vi "sub_PSKMod (User).vi"(0 "Packet to Transmit":i8[](array[numeric]), 2 "PSK system parameters":T2 {"PSK type" items=["normal", "shifted", "offset"]; "symbol map" format="%.3f"}, 7 "Symbol Rate, Hz":dbl=1.0 format="%.2f", 11 "error in (no error)":errorcluster, 12 "filter parameters":T1={"Alpha"=0.5, "Filter Length"=6, "TX Filter"=enum."Root Raised Cos"} {"Alpha" format="%.2f"}) -> (4 "output complex waveform":cluster{"t0":dbl, "dt":dbl, "Y":cdb[]} {"Y" format="%.3f"; "dt" format="%^.2e"; "t0" format="%.4f"}, 8 "samples per symbol":i32, 15 "error out":errorcluster)   [LabVIEW 2013]
uses:
  <vilib>/addons/Modulation/niDMT.lvlib
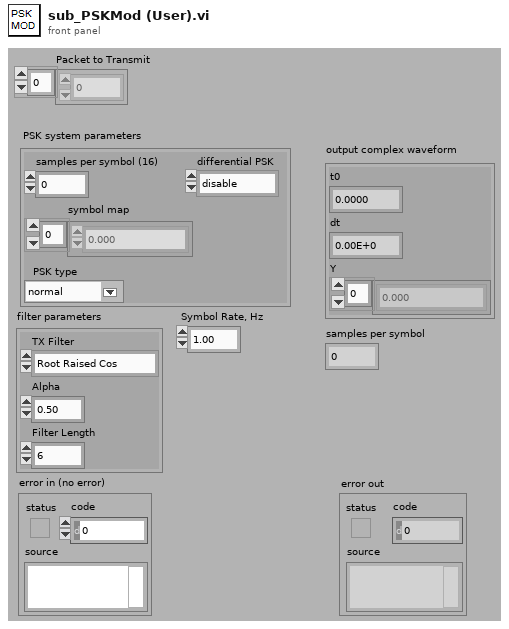
[diagram p1: front panel]
types:
  T1 = cluster{"Alpha":dbl, "Filter Length":i32, "TX Filter":enum16{"none", "Raised Cosine", "Root Raised Cos", "Gaussian"}}
  T2 = cluster{"samples per symbol (16)":i32, "symbol map":cdb[], "differential PSK":enum16{"disable", "enable"}, "PSK type":u16}
  T3 = enum16{"FSK", "PSK", "QAM", "MSK", "PAM", "ASK", "CPM"}
  T4 = enum16{"none", "Raised Cosine", "Root Raised Cos", "Gaussian"}
  T5 = typedef "niAMT.lvlib/Complex Data Waveform.ctl" = cluster{"t0":dbl, "dt":dbl, "Y":cdb[]}
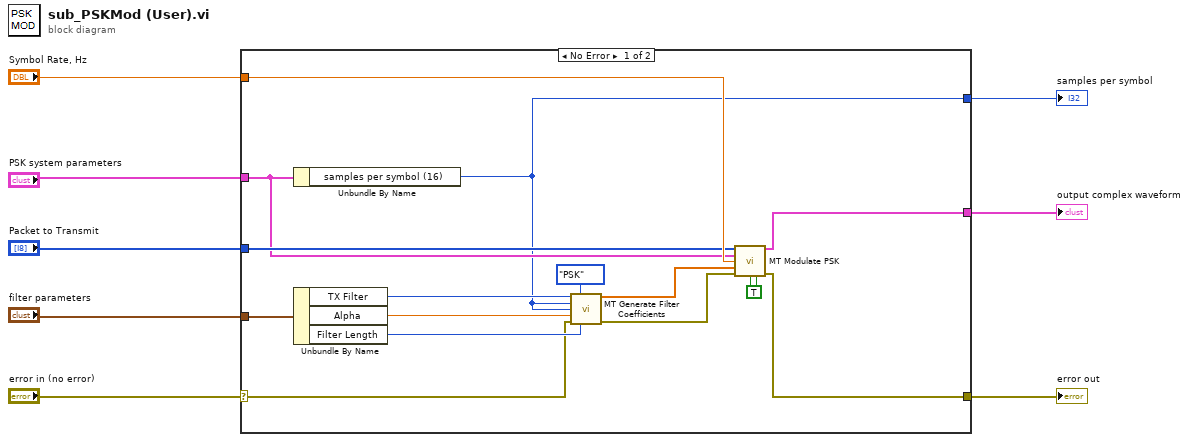
[diagram p0: block diagram]
diagram:
  n1 = case shown="No Error" "error in (no error)" {
    selector: "error in (no error)" -> [w14 w24]
    tunnel: "Symbol Rate, Hz" -> [w22 _]
    tunnel: "PSK system parameters" -> [w12 _]
    tunnel: "filter parameters" -> [w21 _]
    tunnel: "Packet to Transmit" -> [w16 _]
    tunnel: [w11 _] -> w3
    tunnel: [w10 _] -> w2
    tunnel: [w9 w24] -> w1
    frame No Error {
      w23 = TRUE ("Reset (T)")
      n2 = Unbundle By Name(w12) -> ("samples per symbol (16)"=w10:i32)
      n3 = Unbundle By Name(w21) -> ("TX Filter"=w17:T4, "Alpha"=w18:dbl, "Filter Length"=w19:i32)
      n4 = call <vilib>:"MT Generate Filter Coefficients.vi"("pulse shaping filter (none)"=w17, "modulation type"=T3."PSK", "pulse shaping samples per symbol (16)"=w10, "matched samples per symbol (16)"=w10, "filter parameter"=w18, "error in (no error)"=w14, "filter length (symbols)"=w19) -> ("pulse shaping filter coefficients"=w15:dbl[], "error out"=w13:errorcluster)  [unwired: 6 in, 1 out]
      n5 = call <vilib>:"MT Modulate PSK.vi"("input bit stream"=w16, "PSK system parameters"=w12, "symbol rate (Hz)"=w22, "pulse shaping filter coefficients"=w15, "error in (no error)"=w13, "reset? (T)"=w23, "flush buffers? (F)"=w23) -> ("output complex waveform"=w11:T5, "error out"=w9:errorcluster)  [unwired: 6 in, 1 out]
    }
    frame Error {
    }
  }
  "error out" <- w1
  "output complex waveform" <- w3
  "samples per symbol" <- w2
